vi "_Func_array2D_vcmd_vna_wmg.vi"(9 "mode2":T1, 10 "mode1":T3, 11 "mode":string(combo)) -> (2 "clus_mode2":T2, 3 "array2D_mode1":string[][](array[string]))   [LabVIEW 2011]
panel:
  in  "separ_symb_col":string="@"
  in  "separ_symb_row":string="$"
  in  "input_String":string
  in  "separ_symb2":string
  in  "separ_symb1":string
  in  "input_2d":string[][](array[string])
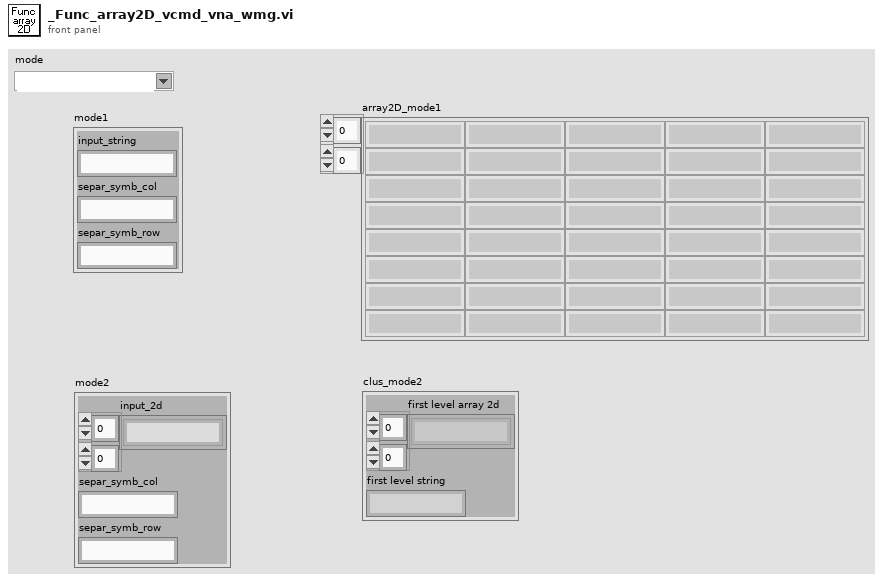
[diagram p1: front panel]
types:
  T1 = cluster{"input_2d":string[][], "separ_symb_col":string, "separ_symb_row":string}
  T2 = cluster{"first level array 2d":string[][], "first level string":string}
  T3 = cluster{"input_string":string, "separ_symb_col":string, "separ_symb_row":string}
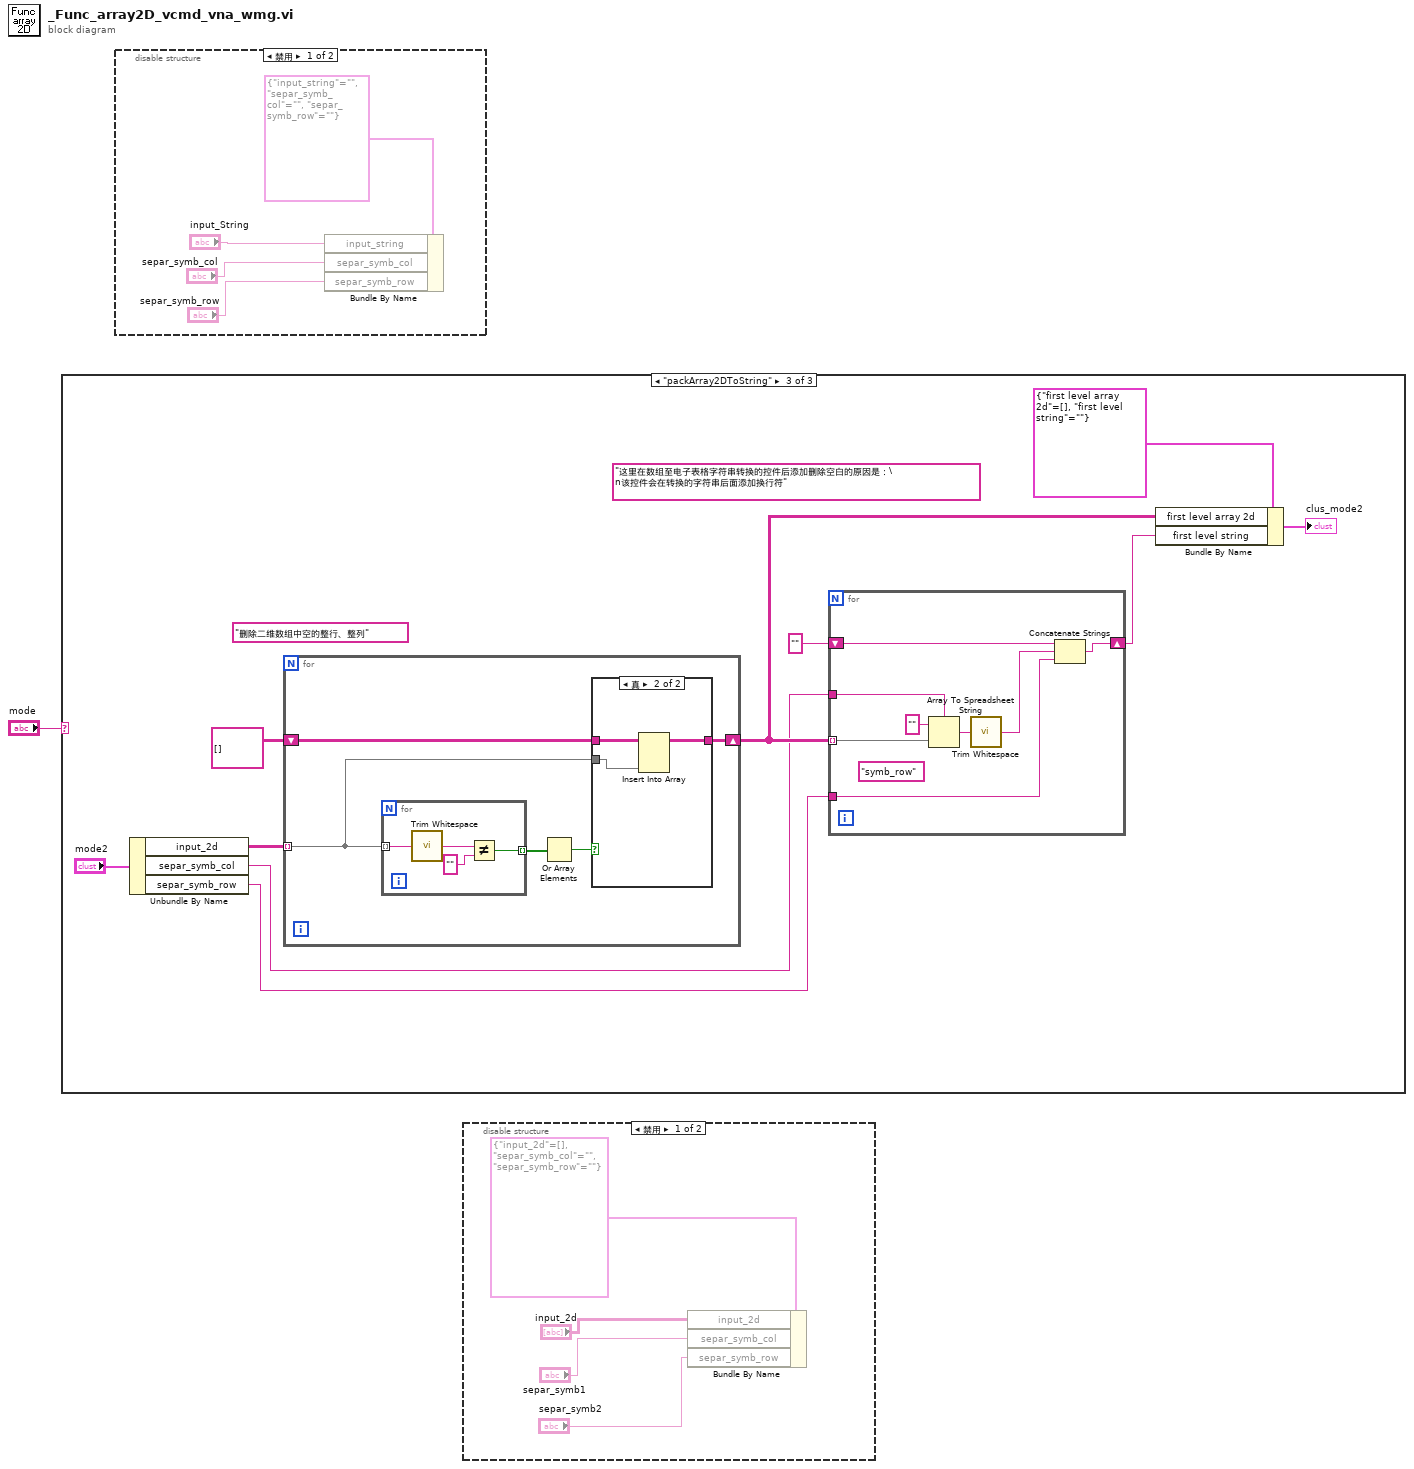
[diagram p0: block diagram]
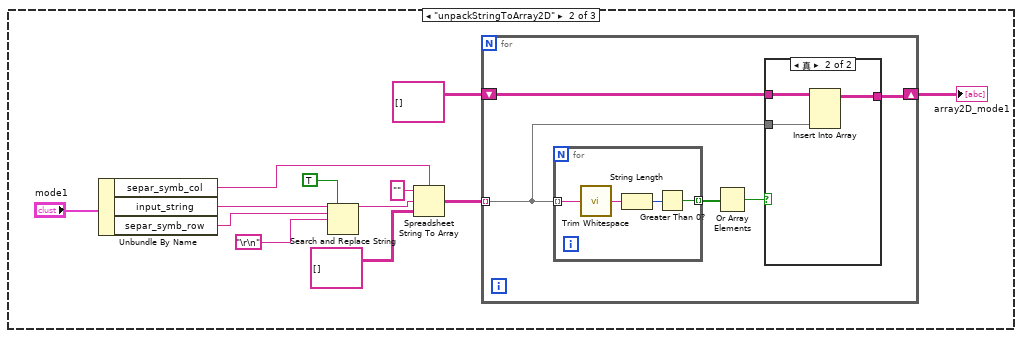
[diagram p5: hidden frame]
diagram:
  n1 = case shown="\"packArray2DToString\"" "mode" {
    frame Default {
    }
    frame "unpackStringToArray2D" {
      n2 = Unbundle By Name("mode1") -> ("separ_symb_col"=w3:string, "input_string"=w5:string, "separ_symb_row"=w4:string)
      n3 = Search and Replace String(replace all?=TRUE ("替换全部？(F)"), input string=w5, search string=w4, replace string="\r\n") -> (result string=w12:string)  [unwired: 4 in, 3 out]
      n4 = Spreadsheet String To Array(delimiter (Tab)=w3, format string="" ("格式字符串"), spreadsheet string=w12, array type (2D Dbl)=string[][] []) -> (array=w8:string[][])
      n5 = for {
        tunnel: w8 -> [w14] mode=indexing
        shift-right: [w15] -> w2
        shift-left: string[][] [] -> [w16]
        n6 = for {
          tunnel: w14 -> [w26] mode=indexing
          tunnel: [w23] -> w18 mode=indexing
          n7 = call <vilib>:"Trim Whitespace.vi"("string"=w26) -> ("trimmed string"=w25:string)  [unwired: 1 in]
          n8 = String Length(string=w25) -> (length=w24:i32)
          n9 = Greater Than 0?(x=w24) -> (x > 0?=w23:bool)
        }
        n10 = Or Array Elements(Boolean array=w18) -> (logical OR=w17:bool)
        n11 = case shown="真" w17 {
          tunnel: w16 -> [w19 w22]
          tunnel: [w19 w21] -> w15
          tunnel: w14 -> [_ w20]
          frame False {
          }
          frame True {
            n12 = Insert Into Array(array=w22, new element=w20) -> (w21:string[][])  [unwired: 2 in]
          }
        }
      }
      "array2D_mode1" <- w2
    }
    frame "packArray2DToString" {
      (unwired) "这里在数组至电子表格字符串转换的控件后添加删除空白的原因是：\n该控件会在转换的字符串后面添加换行符"
      (unwired) "删除二维数组中空的整行、整列"
      n13 = Unbundle By Name("mode2") -> ("input_2d"=w29:string[][], "separ_symb_col"=w28:string, "separ_symb_row"=w27:string)
      n14 = for {
        tunnel: w29 -> [w45] mode=indexing
        shift-right: [w46] -> w34
        shift-left: string[][] [] -> [w47]
        n15 = for {
          tunnel: w45 -> [w57] mode=indexing
          tunnel: [w54] -> w49 mode=indexing
          n16 = call <vilib>:"Trim Whitespace.vi"("string"=w57) -> ("trimmed string"=w56:string)  [unwired: 1 in]
          n17 = Not Equal?(x=w56, y="") -> (x != y?=w54:bool)
        }
        n18 = Or Array Elements(Boolean array=w49) -> (logical OR=w48:bool)
        n19 = case shown="真" w48 {
          tunnel: w47 -> [w50 w53]
          tunnel: w45 -> [_ w52]
          tunnel: [w50 w51] -> w46
          frame False {
          }
          frame True {
            n20 = Insert Into Array(array=w53, new element=w52) -> (w51:string[][])  [unwired: 2 in]
          }
        }
      }
      n21 = for {
        tunnel: w34 -> [w44] mode=indexing
        shift-right: [w41] -> w32
        shift-left: "" -> [w42]
        tunnel: w28 -> [w37]
        tunnel: w27 -> [w38]
        (unwired) "symb_row"
        n22 = Array To Spreadsheet String(delimiter (Tab)=w37, array=w44, 3:"" ("格式字符串")) -> (spreadsheet string=w40:string)
        n23 = call <vilib>:"Trim Whitespace.vi"("string"=w40) -> ("trimmed string"=w39:string)  [unwired: 1 in]
        n24 = Concatenate Strings(w42, w39, w38) -> (w41:string)
      }
      n25 = Bundle By Name(cluster=T2 {"first level array 2d"=[], "first level string"=""} ("输入簇"), "first level array 2d"=w34, "first level string"=w32) -> (→"clus_mode2":T2)
    }
  }
  n26 = disable-structure shown="禁用" {
    frame Disabled {
      n27 = Bundle By Name(cluster=T3 {"input_string"="", "separ_symb_col"="", "separ_symb_row"=""} ("输入簇"), "input_string"="input_String", "separ_symb_col"="separ_symb_col", "separ_symb_row"="separ_symb_row") -> ()  [unwired: 1 out]
    }
    frame Enabled {
    }
  }
  n28 = disable-structure shown="禁用" {
    frame Disabled {
      n29 = Bundle By Name(cluster=T1 {"input_2d"=[], "separ_symb_col"="", "separ_symb_row"=""}, "input_2d"="input_2d", "separ_symb_col"="separ_symb1", "separ_symb_row"="separ_symb2") -> ()  [unwired: 1 out]
    }
    frame Enabled {
    }
  }
